vi "GetAttributeViBoolean_SA-BP_CP_PS.vi"(8 "error in (no error)":errorcluster {"code" format="%.0x"}, 9 "AttributeID":u32(ring)=1150867 items=["SA_BURST_POWER_IF_GAIN_AUTO_ENABLED "=1150867, "SA_BURST_POWER_IF_GAIN_ENABLED "=1150866, "SA_BURSTPOWER_AVERAGE_ENABLED"=1150206, "SA_BURSTPOWER_BURST_WIDTH_AUTO_ENABLED"=1150194, "SA_BURSTPOWER_DISPLAY_BAR_GRAPH_ENABLED"=1150220, "SA_BURSTPOWER_DISPLAY_MAX_HOLD_ENABLED"=1150221, "SA_BURSTPOWER_DISPLAY_MIN_HOLD_ENABLED"=1150222, "SA_BURSTPOWER_DISPLAY_WINDOWX_AUTO_SCALE_ENABLED"=1150214, "SA_BURSTPOWER_DISPLAY_WINDOWY_AUTO_SCALE_ENABLED"=1150217, "SA_BURSTPOWER_MARKER_COUPLE_ENABLED"=1150244, "SA_BURSTPOWER_MARKER_ENABLED"=1150228, "SA_CHANNEL_POWER_POWER_LIMIT_ENABLED"=1150862, "SA_CHANNEL_POWER_PSD_LIMIT_ENABLED"=1150864, "SA_CHANNELPOWER_AVERAGE_ENABLED"=1150252, "SA_CHANNELPOWER_DETECTOR_TYPE_AUTO_ENABLED"=1150249, "SA_CHANNELPOWER_DISPLAY_BAR_GRAPH_ENABLED"=1150302, "SA_CHANNELPOWER_DISPLAY_WINDOWY_AUTO_SCALE_ENABLED"=1150301, "SA_CHANNELPOWER_FREQUENCY_PHASE_NOISE_OPTION_AUTO_ENABLED"=1150263, "SA_CHANNELPOWER_IF_GAIN_AUTO_ENABLED"=1150660, "SA_CHANNELPOWER_IF_GAIN"=1150659, "SA_CHANNELPOWER_MARKER_COUPLE_ENABLED"=1150279, "SA_CHANNELPOWER_MARKER_ENABLED"=1150282, "SA_CHANNELPOWER_OFFSETFILTER_ENABLED"=1150267, "SA_CHANNELPOWER_SWEEPCOUPLING_RESOLUTION_BANDWIDTH_AUTO_ENABLED"=1150258, "SA_CHANNELPOWER_SWEEPCOUPLING_SWEEP_TIME_AUTO_ENABLED"=1150273, "SA_CHANNELPOWER_SWEEPCOUPLING_VIDEO_BANDWIDTH_AUTO_ENABLED"=1150261, "SA_POWERSTATISTICS_DISPLAY_GAUSSIAN_LINE_ENABLED"=1150318, "SA_POWERSTATISTICS_DISPLAY_REFERENCE_TRACE_ENABLED"=1150338, "SA_POWERSTATISTICS_IF_GAIN_AUTO_ENABLED"=1150664, "SA_POWERSTATISTICS_IF_GAIN"=1150663, "SA_POWERSTATISTICS_MARKER_COUPLE_ENABLED"=1150348, "SA_POWERSTATISTICS_MARKER_ENABLED"=1150350], 11 "instrument handle":refnum<k15>) -> (0 "error out":errorcluster {"code" format="%.0x"}, 2 "AttributeValue":bool, 3 "instrument handle out":refnum<k15>)   [LabVIEW 2009, in "Keysight XSAn.lvlib"]
doc: "Gets a Boolean attribute from the instrument driver.\nThe following Attributes are supported:\n\nSA_BURST_POWER_IF_GAIN_AUTO_ENABLED \nSA_BURST_POWER_IF_GAIN_ENABLED \nSA_BURSTPOWER_AVERAGE_ENABLED\nSA_BURSTPOWER_BURST_WIDTH_AUTO_ENABLED\nSA_BURSTPOWER_DISPLAY_BAR_GRAPH_ENABLED\nSA_BURSTPOWER_DISPLAY_MAX_HOLD_ENABLED\nSA_BURSTPOWER_DISPLAY_MIN_HOLD_ENABLED\nSA_BURSTPOWER_DISPLAY_WINDOWX_AUTO_SCALE_ENABLED\nSA_BURSTPOWER_DISPLAY_WINDOWY_AUTO_SCALE_ENABLED\nSA_BURSTPOWER_MARKER_COUPLE_ENABLED\nSA_BURSTPOWER_MARKER_ENABLED\nSA_CHANNEL_POWER_POWER_LIMIT_ENABLED \nSA_CHANNEL_POWER_PSD_LIMIT_ENABLED \nSA_CHANNELPOWER_AVERAGE_ENABLED\nSA_CHANNELPOWER_DETECTOR_TYPE_AUTO_ENABLED\nSA_CHANNELPOWER_DISPLAY_BAR_GRAPH_ENABLED\nSA_CHANNELPOWER_DISPLAY_WINDOWY_AUTO_SCALE_ENABLED\nSA_CHANNELPOWER_FREQUENCY_PHASE_NOISE_OPTION_AUTO_ENABLED\nSA_CHANNELPOWER_IF_GAIN_AUTO_ENABLED\nSA_CHANNELPOWER_IF_GAIN\nSA_CHANNELPOWER_MARKER_COUPLE_ENABLED\nSA_CHANNELPOWER_MARKER_ENABLED\nSA_CHANNELPOWER_OFFSETFILTER_ENABLED\nSA_CHANNELPOWER_SWEEPCOUPLING_RESOLUTION_BANDWIDTH_AUTO_ENABLED\nSA_CHANNELPOWER_SWEEPCOUPLING_SWEEP_TIME_AUTO_ENABLED\nSA_CHANNELPOWER_SWEEPCOUPLING_VIDEO_BANDWIDTH_AUTO_ENABLED\nSA_POWERSTATISTICS_DISPLAY_GAUSSIAN_LINE_ENABLED\nSA_POWERSTATISTICS_DISPLAY_REFERENCE_TRACE_ENABLED\nSA_POWERSTATISTICS_IF_GAIN_AUTO_ENABLED\nSA_POWERSTATISTICS_IF_GAIN\nSA_POWERSTATISTICS_MARKER_COUPLE_ENABLED\nSA_POWERSTATISTICS_MARKER_ENABLED"
uses:
  <instrlib>/Keysight XSAn/Keysight XSAn.lvlib
  AgXSAn.dll
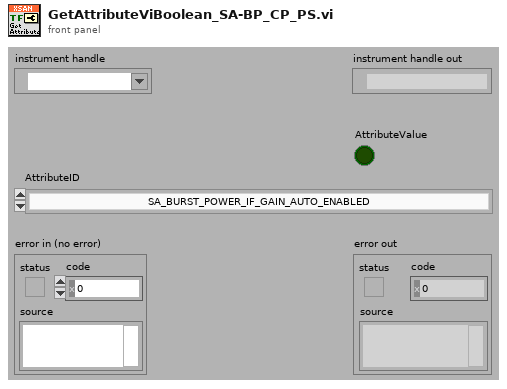
[diagram p1: front panel]
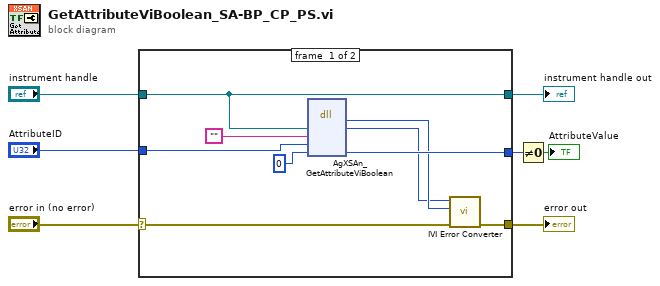
[diagram p0: block diagram]
diagram:
  n1 = case shown="No Error" "error in (no error)" {
    selector: "error in (no error)" -> [w16 w18]
    tunnel: [w15 w18] -> w7
    tunnel: "instrument handle" -> [w11 w17]
    tunnel: "AttributeID" -> [w14 _]
    tunnel: [w12 _] -> w2
    tunnel: [w11 w17] -> w1
    frame #0 {
      n2 = dll-call lib="AgXSAn**.dll" fn="AgXSAn_GetAttributeViBoolean"("Vi"=w11, "RepCapIdentifier"="", "AttributeID"=w14, "AttributeValue"=i16 0) -> ("return type"=w9:i32, "Vi"=w8:u32, "AttributeValue"=w12:i16)  [unwired: 5 in, 2 out]
      n3 = call <instrlib>:"IVI Error Converter.vi"("error in (no error)"=w16, "IVI error code (0)"=w9, "instrument handle"=w8) -> ("error out"=w15:errorcluster)  [unwired: 7 in, 1 out]
    }
    frame #1 {
    }
  }
  "error out" <- w7
  "instrument handle out" <- w1
  n4 = Not Equal To 0?(x=w2) -> (x != 0?=→"AttributeValue":bool)
